vi "Img Json Parser.vi"(8 "error in (no error)":errorcluster, 11 "Json string":string) -> (0 "error out":errorcluster, 2 "found":bool, 3 "Json data":T1)   [LabVIEW 2018, in "Image Json Parser.lvclass"]
uses:
  Image Json Parser.lvclass
  Img Json Data.ctl
  Img Json Frames.ctl
  Img Json Meta.ctl
  e3236b34-dc2b-424c-9cb1-501829c4a3b5.vi
  8fdaca5c-5aa5-44ec-82b8-04d894ecbc62.vi
  <vilib>/JDP Science/JSONtext/Next JSON Value.vi
  <vilib>/JDP Science/JSONtext/String Subset.vi
  <vilib>/JDP Science/JSONtext/Parsing/Advance past next JSON Value (inlined COPY).vi
  <vilib>/JDP Science/JSONtext/Parsing/Advance past whitespace.vi
  <vilib>/JDP Science/JSONtext/Parsing/Advance past String.vi
  <vilib>/JDP Science/JSONtext/Parsing/Advance past Number.vi
  <vilib>/JDP Science/JSONtext/Parsing/Advance past Line Ending.vi
  <vilib>/JDP Science/JSONtext/Parsing/Parse Full Path or Item Name.vi
  <vilib>/JDP Science/JSONtext/Parsing/Advance past Array.vi
  <vilib>/JDP Science/JSONtext/Parsing/Advance past Object.vi
  <vilib>/JDP Science/JSONtext/support/Error Cluster From Code.vi
  <vilib>/JDP Science/JSONtext/Offset/Find Item Locations by Path.vi
  <vilib>/JDP Science/JSONtext/JSON text to Variant.vi
  <vilib>/JDP Science/JSONtext/LVClass Serializer/JSONtext LVClass Serializer.lvclass
  <vilib>/JDP Science/JSONtext/JSONtext.lvlib
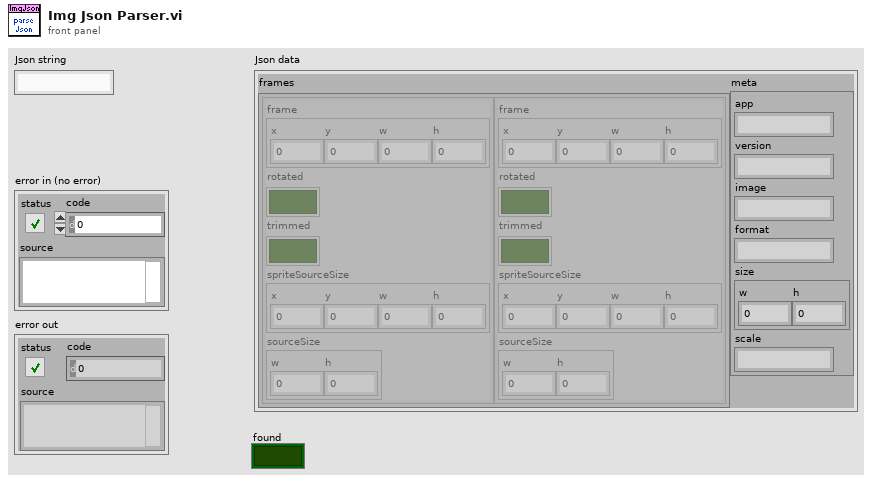
[diagram p1: front panel]
types:
  T1 = typedef "Image Json Parser.lvclass/Img Json Data.ctl" = cluster{"frames":T2[], "meta":T3}
  T2 = typedef "Image Json Parser.lvclass/Img Json Frames.ctl" = cluster{"frame":cluster{"x":i32, "y":i32, "w":i32, "h":i32}, "rotated":bool, "trimmed":bool, "spriteSourceSize":cluster{"x":i32, "y":i32, "w":i32, "h":i32}, "sourceSize":cluster{"w":i32, "h":i32}}
  T3 = typedef "Image Json Parser.lvclass/Img Json Meta.ctl" = cluster{"app":string, "version":string, "image":string, "format":string, "size":cluster{"w":i32, "h":i32}, "scale":string}
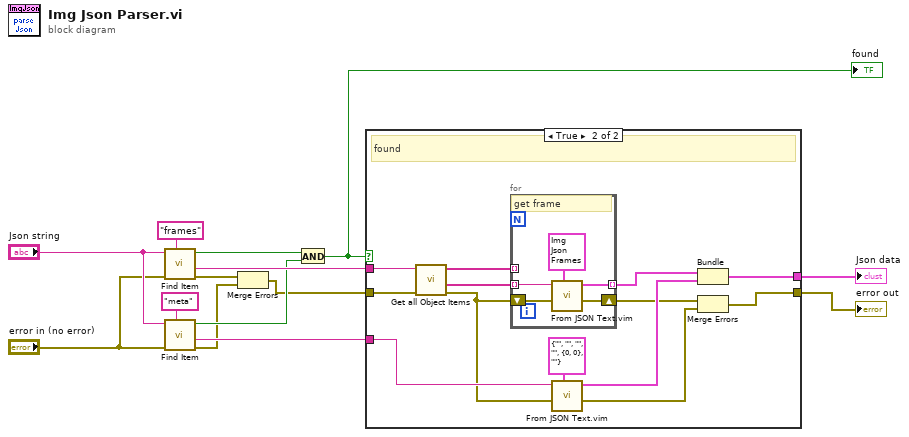
[diagram p0: block diagram]
diagram:
  n1 = call <vilib>:"Find Item.vi"("$Path or Item Name"="frames", "error in (no error)"="error in (no error)", "JSON"="Json string") -> ("error out"=w5:errorcluster, "<JSON>"=w13:string, "Found"=w9:bool)  [unwired: 5 in, 1 out]
  n2 = call <vilib>:"Find Item.vi"("$Path or Item Name"="meta", "error in (no error)"="error in (no error)", "JSON"="Json string") -> ("error out"=w4:errorcluster, "<JSON>"=w7:string, "Found"=w10:bool)  [unwired: 5 in, 1 out]
  n3 = Merge Errors(w5, w4) -> (w3:errorcluster)
  n4 = And(x=w9, y=w10) -> (x .and. y?=w8:bool)
  "found" <- w8
  n5 = case shown="True" w8 {
    tunnel: w13 -> [_ w28]
    tunnel: w7 -> [_ w25]
    tunnel: [_ w21] -> w6
    tunnel: w3 -> [w15 w20]
    tunnel: [w15 w16] -> w1
    frame False {
    }
    frame True {
      # "found"
      n6 = call <vilib>:"Get all Object Items.vi"("error in (no error)"=w20, "JSON"=w28) -> ("error out"=w19:errorcluster, "<JSON>"=w27:string[], "Item Names"=w26:string[])  [unwired: 6 in, 1 out]
      n7 = for {
        tunnel: w27 -> [w33] mode=indexing
        tunnel: w26 -> [_] mode=indexing
        tunnel: [w31] -> w23 mode=indexing
        shift-right: [w29] -> w18
        shift-left: w19 -> [w30]
        # "get frame"
        n8 = call "From JSON Text.vim"("Data Type and Default Value"=T2 {"frame"={"x"=0, "y"=0, "w"=0, "h"=0}, "rotated"=FALSE, "trimmed"=FALSE, "spriteSourceSize"={"x"=0, "y"=0, "w"=0, "h"=0}, "sourceSize"={"w"=0, "h"=0}} ("frames"), "error in (no error)"=w30, "JSON"=w33) -> ("error out"=w29:errorcluster, "Data out"=w31:T2)  [unwired: 7 in]
      }
      n9 = call "From JSON Text.vim"("Data Type and Default Value"=T3 {"app"="", "version"="", "image"="", "format"="", "size"={"w"=0, "h"=0}, "scale"=""} ("meta"), "error in (no error)"=w19, "JSON"=w25) -> ("error out"=w17:errorcluster, "Data out"=w22:T3)  [unwired: 7 in]
      n10 = Bundle(w23, "Data out"=w22) -> (w21:cluster{T2[], "Data out":T3})  [unwired: 1 in]
      n11 = Merge Errors(w18, w17) -> (w16:errorcluster)
    }
  }
  "Json data" <- w6
  "error out" <- w1
